vi "CRYHarmonic curves x-axis replace.vi"(10 "New X axis":dbl[](array[numeric]) format="%.2f", 11 "Freq resp curves":cluster{cluster{"x":dbl, "y":dbl, "z":dbl}[]}[](array[cluster]) {"?"."z" format="%.2f"; "?"."y" format="%.2f"; "?"."x" format="%.2f"}) -> (3 "Freq resp curves out":cluster{cluster{"x":dbl, "y":dbl, "z":dbl}[]}[](array[cluster]) {"?"."z" format="%.2f"; "?"."y" format="%.2f"; "?"."x" format="%.2f"})   [LabVIEW 2013]
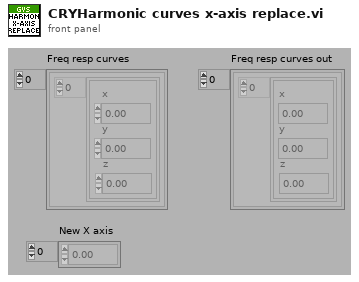
[diagram p1: front panel]
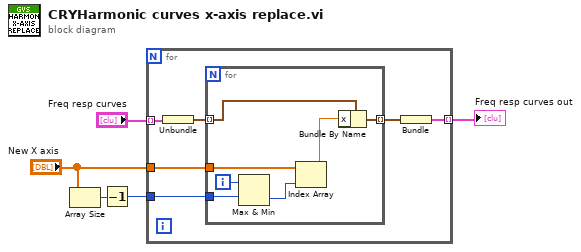
[diagram p0: block diagram]
diagram:
  n1 = Array Size(array="New X axis") -> (size(s)=w2:i32)
  n2 = Decrement(x=w2) -> (x-1=w1:i32)
  n3 = for {
    tunnel: "Freq resp curves" -> [w11] mode=indexing
    tunnel: [w8] -> w4 mode=indexing
    tunnel: "New X axis" -> [w7]
    tunnel: w1 -> [w6]
    n4 = Unbundle(w11) -> (w10:cluster{"x":dbl, "y":dbl, "z":dbl}[])
    n5 = for {
      tunnel: w10 -> [w18] mode=indexing
      tunnel: [w17] -> w9 mode=indexing
      tunnel: w7 -> [w14]
      tunnel: w6 -> [w16]
      i -> [w15]
      n6 = Max & Min(x=w15, y=w16) -> (min(x,y)=w13:i32)  [unwired: 1 out]
      n7 = Index Array(array=w14, index=w13) -> (element=w12:dbl)
      n8 = Bundle By Name(cluster=w18, "x"=w12) -> (w17:cluster{"x":dbl, "y":dbl, "z":dbl})
    }
    n9 = Bundle(w9) -> (w8:cluster{cluster{"x":dbl, "y":dbl, "z":dbl}[]})  [unwired: 1 in]
  }
  "Freq resp curves out" <- w4
